vi "Operaciones Matematicas.vi"() -> ()   [LabVIEW 2022 SP3]
panel:
  out "Area":dbl format="%#_3f"
  in  "Semi eje menor(b)":dbl(knob) scale=0.0..500.0
  in  "Semi eje mayo(a)":dbl(knob) scale=0.0..500.0
  out "Resultado":dbl
  in  "Variable B":dbl
  in  "Varible A":dbl
  # "Operaciones matematicas con labview"
  # "Elipse"
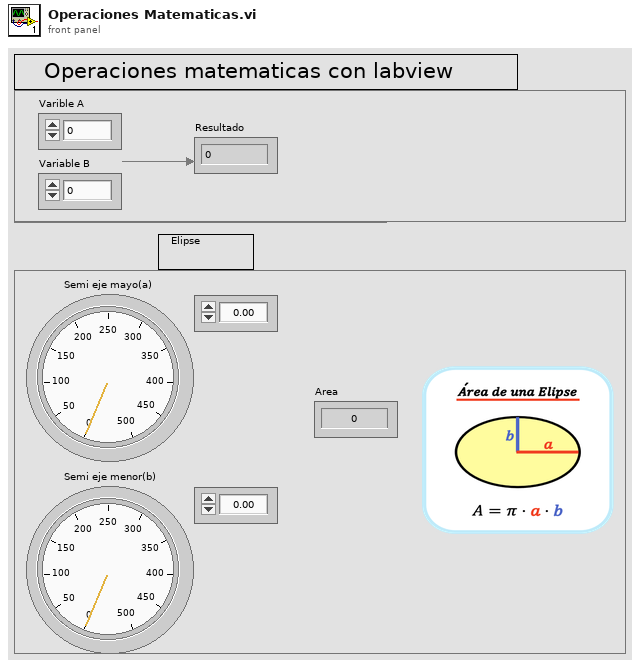
[diagram p1: front panel]
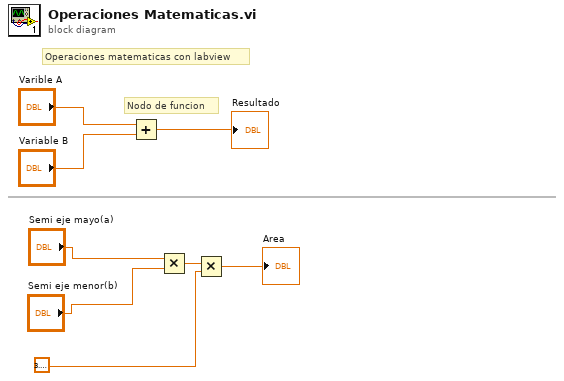
[diagram p0: block diagram]
diagram:
  # "Nodo de funcion"
  # "Operaciones matematicas con labview"
  n1 = Add(x="Varible A", y="Variable B") -> (x+y=→"Resultado":dbl)
  n2 = Multiply(x="Semi eje mayo(a)", y="Semi eje menor(b)") -> (x*y=w3:dbl)
  n3 = Multiply(x=w3, y=3.141592653589793) -> (x*y=→"Area":dbl)
